vi "RBF Graph.vi"(4 "STD":dbl, 6 "Number":i32, 7 "Array of Double 3":dbl[](array[numeric]), 9 "x_f":dbl, 10 "x_0":dbl, 11 "Number 2":i32) -> (3 "Array":cluster{dbl[], dbl[]}[](array[cluster]))   [LabVIEW 2021]
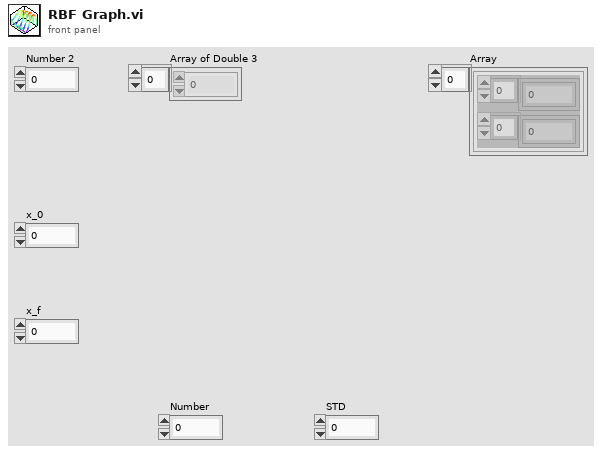
[diagram p1: front panel]
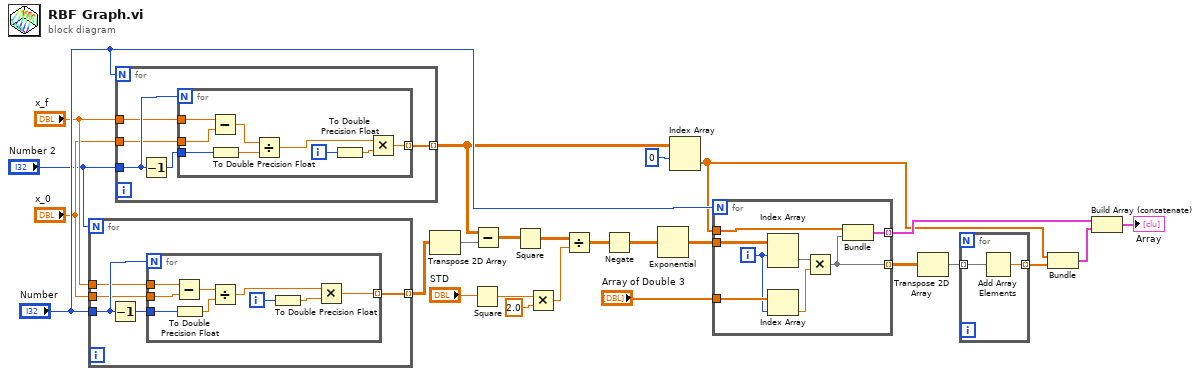
[diagram p0: block diagram]
diagram:
  n1 = for {
    N: "Number 2" -> [_]
    tunnel: [w29] -> w12 mode=indexing
    tunnel: "Number" -> [w28]
    tunnel: "x_f" -> [w27]
    tunnel: "x_0" -> [w26]
    n2 = Decrement(x=w28) -> (x-1=w30:i32)
    n3 = for {
      N: w28 -> [_]
      tunnel: w27 -> [w39]
      tunnel: w26 -> [w37]
      tunnel: [w38] -> w29 mode=indexing
      tunnel: w30 -> [w34]
      i -> [w32]
      n4 = Subtract(x=w39, y=w37) -> (x-y=w36:dbl)
      n5 = To Double Precision Float(number=w34) -> (double precision float=w33:dbl)
      n6 = Divide(x=w36, y=w33) -> (x/y=w35:dbl)
      n7 = To Double Precision Float(number=w32) -> (double precision float=w31:dbl)
      n8 = Multiply(x=w35, y=w31) -> (x*y=w38:dbl)
    }
  }
  n9 = for {
    N: "Number" -> [_]
    tunnel: [w43] -> w5 mode=indexing
    tunnel: "Number 2" -> [w42]
    tunnel: "x_f" -> [w41]
    tunnel: "x_0" -> [w40]
    n10 = Decrement(x=w42) -> (x-1=w44:i32)
    n11 = for {
      N: w42 -> [_]
      tunnel: w41 -> [w53]
      tunnel: w40 -> [w51]
      tunnel: [w52] -> w43 mode=indexing
      tunnel: w44 -> [w48]
      i -> [w45]
      n12 = Subtract(x=w53, y=w51) -> (x-y=w50:dbl)
      n13 = To Double Precision Float(number=w48) -> (double precision float=w47:dbl)
      n14 = Divide(x=w50, y=w47) -> (x/y=w49:dbl)
      n15 = To Double Precision Float(number=w45) -> (double precision float=w46:dbl)
      n16 = Multiply(x=w49, y=w46) -> (x*y=w52:dbl)
    }
  }
  n17 = Transpose 2D Array(2D array=w12) -> (transposed array=w11:dbl[][])
  n18 = Square(x="STD") -> (x^2=w21:dbl)
  n19 = Subtract(x=w5, y=w11) -> (x-y=w17:dbl[][])
  n20 = Square(x=w17) -> (x^2=w16:dbl[][])
  n21 = Multiply(x=w21, y=2.0) -> (x*y=w24:dbl)
  n22 = Divide(x=w16, y=w24) -> (x/y=w15:dbl[][])
  n23 = Negate(x=w15) -> (-x=w14:dbl[][])
  n24 = Exponential(1:w14) -> (0:w2:dbl[][])
  n25 = Index Array(array=w5, index (row)=0) -> (element=w3:dbl[])  [unwired: 1 in]
  n26 = for {
    N: "Number" -> [_]
    tunnel: w2 -> [w61]
    tunnel: [w60] -> w8 mode=indexing
    tunnel: "Array of Double 3" -> [w59]
    tunnel: w3 -> [w55]
    tunnel: [w54] -> w1 mode=indexing
    i -> [w58]
    n27 = Index Array(array=w61, index (row)=w58) -> (element=w56:dbl[])  [unwired: 1 in]
    n28 = Index Array(array=w59, index=w58) -> (element=w57:dbl)
    n29 = Multiply(x=w56, y=w57) -> (x*y=w54:dbl[])
    n30 = Bundle(w55, w54) -> (w60:cluster{dbl[], dbl[]})  [unwired: 1 in]
  }
  n31 = Transpose 2D Array(2D array=w1) -> (transposed array=w10:dbl[][])
  n32 = for {
    tunnel: w10 -> [w63] mode=indexing
    tunnel: [w62] -> w9 mode=indexing
    n33 = Add Array Elements(numeric array=w63) -> (sum=w62:dbl)
  }
  n34 = Bundle(w3, w9) -> (w6:cluster{dbl[], dbl[]})  [unwired: 1 in]
  n35 = Build Array (concatenate)(w8, w6) -> (→"Array":cluster{dbl[], dbl[]}[])
